vi "FPGA_main_sensorTest.vi"() -> ()   [LabVIEW 2020]
doc: "256-pt. MA filter in AI chain with control effort linearization based on feedback position."
uses:
  <vilib>/rvi/Emulation/niFpgaGetClockAttributes.vi
  <vilib>/rvi/Emulation/niFpgaSctlEmulationGetInTimedLoop.vi
  <vilib>/rvi/Emulation/niFpgaEmulationReportErrorSimple.vi
  <vilib>/rvi/eio/common/nirviEmuTemplateMethod_errors.vi
  <vilib>/rvi/Emulation/niFpgaEmulationIsFPGAContextNoSignature.vi
  <vilib>/rvi/errors/niFpgaSetErrorForExecOnDevCompSimple.vi
  <vilib>/rvi/eio/common/nirviEmuReportErrorAndStop.vi
  <vilib>/rvi/DataTransferAndStorage/Container/Common/niFpgaContainerGetUniqueNameForEmu.vi
  <vilib>/rvi/FIFO/Fifo_Resource/nirvififoEmulationSetSize.vi
  <vilib>/rvi/FIFO/Fifo_Resource/nirviFifoEmulationQueueMgr.vi
  <instcachedir>/0/nirviFifoEmulationQueueMgr_E5CAEC123FF24DC58D834DCA3CDAA9B5.lvgen/nirviFifoEmulationQueueMgr_E5CAEC123FF24DC58D834DCA3CDAA9B5_001.vi
  <vilib>/rvi/FIFO/Fifo_Resource/nirvififoEmulationDetermineInputValidOut.vi
  <vilib>/rvi/FIFO/Fifo_Resource/nirvififoEmulationCreateLock.vi
  <vilib>/rvi/Emulation/niFpgaProcessEmulError.vi
  <vilib>/rvi/FIFO/Fifo_Resource/nirvififoEmulationObtainLock.vi
  <vilib>/rvi/FIFO/Fifo_Resource/nirvififoEmulationReleaseLock.vi
  <vilib>/rvi/occurrence/nirviWaitOnOccurrenceBase.vi
  <vilib>/rvi/errors/nirviReportUnexpectedCaseInternalError.vi
  <vilib>/rvi/errors/nirviReportUnexpectedCaseInternalError (U32).vi
  <vilib>/rvi/Emulation/niFpgaCriticalErrorInLSC.vi
  <vilib>/Utility/error.llb/Clear Errors.vi
  <vilib>/eio/EIONode/EIONode.xnode
  <vilib>/rvi/DataTransferAndStorage/Container/XNode/niFpgaContainer.xnode
  <vilib>/rvi/FIFO/Fifo_Resource/nirvififoEmulationWrite.vi
  <vilib>/rvi/FIFO/Fifo_Resource/nirvififoEmulationRead.vi
  Components/FPGA functions/FPGA functions.lvlib
panel:
  out "AI LS filter Loop time [us]":u8
  out "Mod7 (NI 9222) AI":fxp<+/-,25,5>[](array[numeric])
  out "AI LS Loop time [us]":u8
  out "FPGA AI LS FIFO\nOverflow?":bool
  out "Mod8 (NI 9222) AI":fxp<+/-,25,5>[](array[numeric])
  out "AI HS filter Loop time [ticks]":u8
  out "FPGA AI HS FIFO\nOverflow?":bool
  out "AI HS Loop time [ticks]":u8
  # "1 tick = 25 ns"
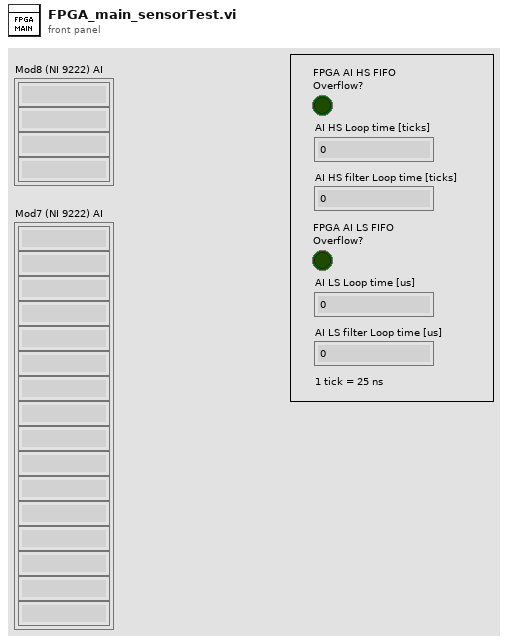
[diagram p1: front panel]
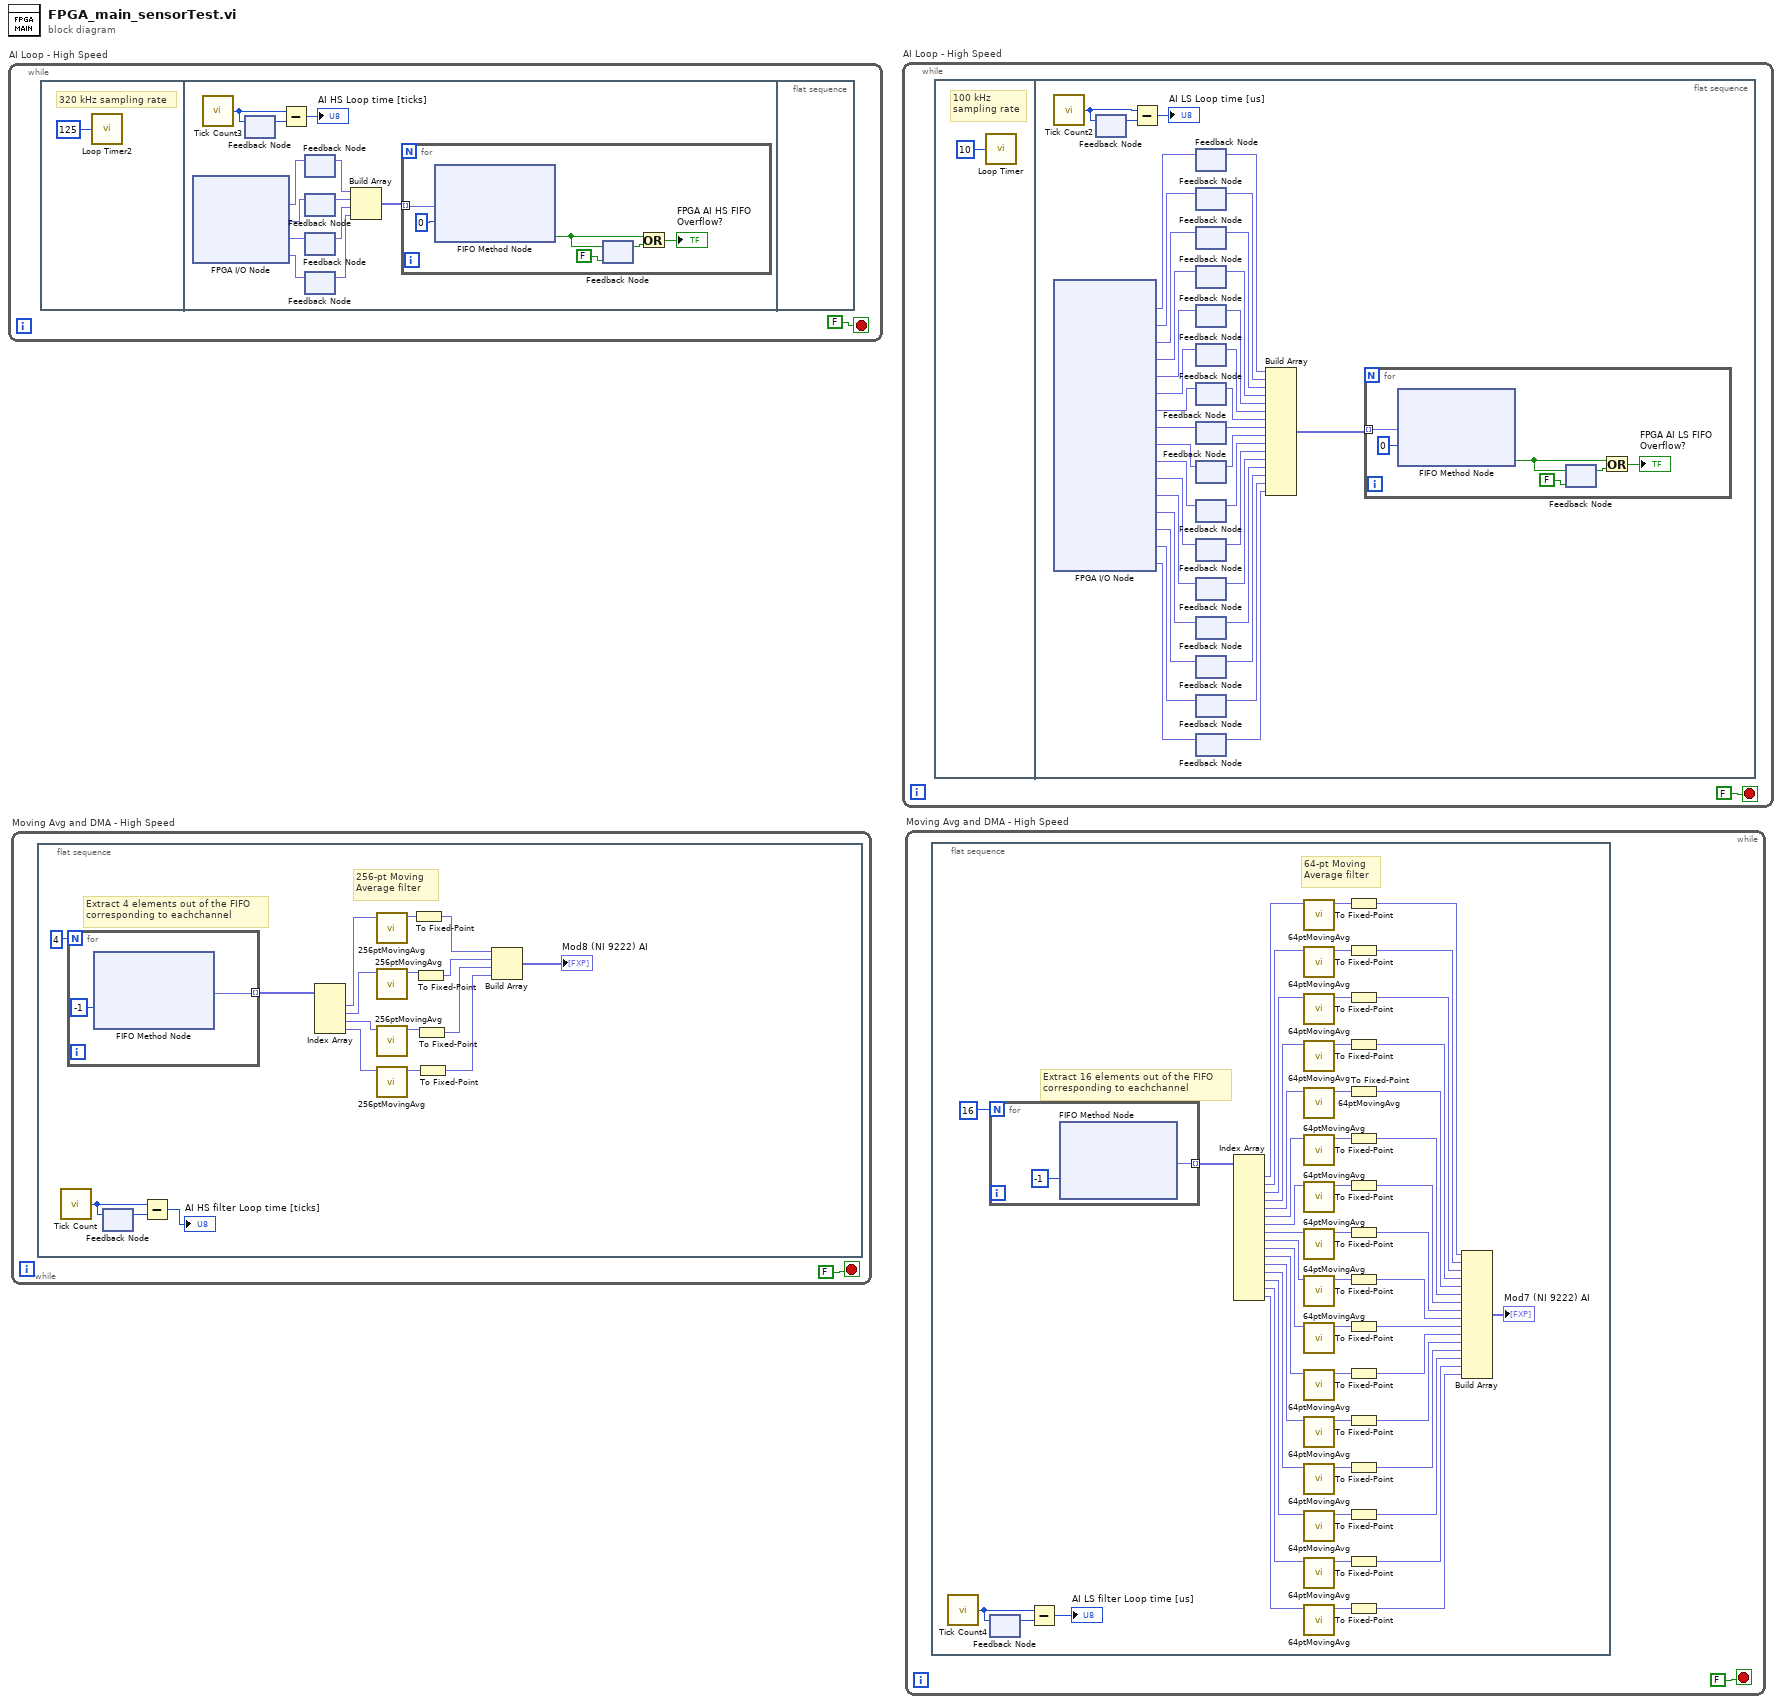
[diagram p0: block diagram]
diagram:
  n1 = while "AI Loop - High Speed" {
    stop <- FALSE stop-if-true
    n2 = flat-sequence {
      frame #0 {
        # "320 kHz sampling rate"
        n3 = call "Loop Timer2"("Count(Ticks)"=u8 125) -> ()  [unwired: 1 out]
      }
      frame #1 {
        n4 = xnode "FPGA I/O Node"() -> ("Mod8/AI0"=w9:fxp<+/-,24,5>, "Mod8/AI1"=w8:fxp<+/-,24,5>, "Mod8/AI2"=w7:fxp<+/-,24,5>, "Mod8/AI3"=w6:fxp<+/-,24,5>)  [unwired: 4 in, 4 out]
        n5 = call "Tick Count3"() -> ("Tick Count(Ticks)"=w14:u8)
        n6 = feedback #1() -> (w13:u8)  [unwired: 1 in]
        n7 = feedback-in #1(w14) -> ()
        n8 = Subtract(x=w14, y=w13) -> (x-y=→"AI HS Loop time [ticks]":u8)
        n9 = feedback-in #2(w9) -> ()
        n10 = feedback #2() -> (w10:fxp<+/-,24,5>)  [unwired: 1 in]
        n11 = feedback #3() -> (w5:fxp<+/-,24,5>)  [unwired: 1 in]
        n12 = feedback-in #3(w8) -> ()
        n13 = feedback #4() -> (w4:fxp<+/-,24,5>)  [unwired: 1 in]
        n14 = feedback-in #4(w7) -> ()
        n15 = feedback #5() -> (w3:fxp<+/-,24,5>)  [unwired: 1 in]
        n16 = feedback-in #5(w6) -> ()
        n17 = Build Array(w10, w5, w4, w3) -> (w11:fxp<+/-,24,5>[])
        n18 = for {
          tunnel: w11 -> [w19] mode=indexing
          n19 = xnode ("FIFO Method Node")("Element"=w19, "Timeout"=0) -> ("Timed Out?"=w16:bool)  [unwired: 1 in, 1 out]
          n20 = feedback-in #6(w16) -> ()
          n21 = feedback #6(FALSE ("Timed Out?")) -> (w17:bool)
          n22 = Or(x=w16, y=w17) -> (x .or. y?=→"FPGA AI HS FIFO\nOverflow?":bool)
        }
      }
      frame #2 {
      }
    }
  }
  n23 = while "Moving Avg and DMA - High Speed" {
    stop <- FALSE stop-if-true
    n24 = flat-sequence {
      frame #0 {
        # "256-pt Moving \nAverage filter"
        # "Extract 4 elements out of the FIFO \ncorresponding to eachchannel"
        n25 = call "Tick Count"() -> ("Tick Count(Ticks)"=w38:u8)
        n26 = for {
          N: 4 -> [_]
          tunnel: [w40] -> w35 mode=indexing
          n27 = xnode ("FIFO Method Node")("Timeout"=-1) -> ("Element"=w40:fxp<+/-,24,5>)  [unwired: 1 in, 2 out]
        }
        n28 = feedback #7() -> (w37:u8)  [unwired: 1 in]
        n29 = feedback-in #7(w38) -> ()
        n30 = Subtract(x=w38, y=w37) -> (x-y=→"AI HS filter Loop time [ticks]":u8)
        n31 = Index Array(array=w35) -> (element #1=w34:fxp<+/-,24,5>, element #2=w33:fxp<+/-,24,5>, element #3=w31:fxp<+/-,24,5>, element #4=w32:fxp<+/-,24,5>)  [unwired: 4 in]
        n32 = call "256ptMovingAvg.vi"("Raw input"=w34) -> ("Output"=w30:fxp<+/-,28,5>)  [unwired: 10 in]
        n33 = call "256ptMovingAvg.vi"("Raw input"=w33) -> ("Output"=w28:fxp<+/-,28,5>)  [unwired: 10 in]
        n34 = call "256ptMovingAvg.vi"("Raw input"=w31) -> ("Output"=w27:fxp<+/-,28,5>)  [unwired: 10 in]
        n35 = call "256ptMovingAvg.vi"("Raw input"=w32) -> ("Output"=w24:fxp<+/-,28,5>)  [unwired: 10 in]
        n36 = To Fixed-Point(number=w30) -> (fixed-point=w29:fxp<+/-,25,5>)  [unwired: 1 in]
        n37 = To Fixed-Point(number=w28) -> (fixed-point=w26:fxp<+/-,25,5>)  [unwired: 1 in]
        n38 = To Fixed-Point(number=w27) -> (fixed-point=w25:fxp<+/-,25,5>)  [unwired: 1 in]
        n39 = To Fixed-Point(number=w24) -> (fixed-point=w23:fxp<+/-,25,5>)  [unwired: 1 in]
        n40 = Build Array(w29, w26, w25, w23) -> (→"Mod8 (NI 9222) AI":fxp<+/-,25,5>[])
      }
    }
  }
  n41 = while "AI Loop - High Speed" {
    stop <- FALSE stop-if-true
    n42 = flat-sequence {
      frame #0 {
        # "100 kHz \nsampling rate"
        n43 = call "Loop Timer"("Count(uSec)"=u8 10 ("Count(Ticks)")) -> ()  [unwired: 1 out]
      }
      frame #1 {
        n44 = call "Tick Count2"() -> ("Tick Count(uSec)"=w79:u8)
        n45 = xnode "FPGA I/O Node"() -> ("Mod7/AI0"=w75:fxp<+/-,24,5>, "Mod7/AI1"=w74:fxp<+/-,24,5>, "Mod7/AI2"=w73:fxp<+/-,24,5>, "Mod7/AI3"=w72:fxp<+/-,24,5>, "Mod7/AI4"=w71:fxp<+/-,24,5>, "Mod7/AI5"=w70:fxp<+/-,24,5>, "Mod7/AI6"=w69:fxp<+/-,24,5>, "Mod7/AI7"=w68:fxp<+/-,24,5>, "Mod7/AI8"=w67:fxp<+/-,24,5>, "Mod7/AI9"=w66:fxp<+/-,24,5>, "Mod7/AI10"=w65:fxp<+/-,24,5>, "Mod7/AI11"=w64:fxp<+/-,24,5>, "Mod7/AI12"=w63:fxp<+/-,24,5>, "Mod7/AI13"=w62:fxp<+/-,24,5>, "Mod7/AI14"=w61:fxp<+/-,24,5>, "Mod7/AI15"=w60:fxp<+/-,24,5>)  [unwired: 16 in, 16 out]
        n46 = feedback #8() -> (w78:u8)  [unwired: 1 in]
        n47 = feedback-in #8(w79) -> ()
        n48 = Subtract(x=w79, y=w78) -> (x-y=→"AI LS Loop time [us]":u8)
        n49 = feedback #9() -> (w59:fxp<+/-,24,5>)  [unwired: 1 in]
        n50 = feedback-in #9(w75) -> ()
        n51 = feedback #10() -> (w58:fxp<+/-,24,5>)  [unwired: 1 in]
        n52 = feedback-in #10(w74) -> ()
        n53 = feedback #11() -> (w57:fxp<+/-,24,5>)  [unwired: 1 in]
        n54 = feedback-in #11(w73) -> ()
        n55 = feedback #12() -> (w56:fxp<+/-,24,5>)  [unwired: 1 in]
        n56 = feedback-in #12(w72) -> ()
        n57 = feedback #13() -> (w55:fxp<+/-,24,5>)  [unwired: 1 in]
        n58 = feedback-in #13(w71) -> ()
        n59 = feedback #14() -> (w54:fxp<+/-,24,5>)  [unwired: 1 in]
        n60 = feedback-in #14(w70) -> ()
        n61 = feedback #15() -> (w53:fxp<+/-,24,5>)  [unwired: 1 in]
        n62 = feedback-in #15(w69) -> ()
        n63 = feedback #16() -> (w52:fxp<+/-,24,5>)  [unwired: 1 in]
        n64 = feedback-in #16(w68) -> ()
        n65 = feedback #17() -> (w51:fxp<+/-,24,5>)  [unwired: 1 in]
        n66 = feedback-in #17(w67) -> ()
        n67 = feedback #18() -> (w50:fxp<+/-,24,5>)  [unwired: 1 in]
        n68 = feedback-in #18(w66) -> ()
        n69 = feedback #19() -> (w49:fxp<+/-,24,5>)  [unwired: 1 in]
        n70 = feedback-in #19(w65) -> ()
        n71 = feedback #20() -> (w48:fxp<+/-,24,5>)  [unwired: 1 in]
        n72 = feedback-in #20(w64) -> ()
        n73 = feedback #21() -> (w47:fxp<+/-,24,5>)  [unwired: 1 in]
        n74 = feedback-in #21(w63) -> ()
        n75 = feedback #22() -> (w46:fxp<+/-,24,5>)  [unwired: 1 in]
        n76 = feedback-in #22(w62) -> ()
        n77 = feedback #23() -> (w45:fxp<+/-,24,5>)  [unwired: 1 in]
        n78 = feedback-in #23(w61) -> ()
        n79 = feedback #24() -> (w44:fxp<+/-,24,5>)  [unwired: 1 in]
        n80 = feedback-in #24(w60) -> ()
        n81 = Build Array(w59, w58, w57, w56, w55, w54, w53, w52, w51, w50, w49, w48, w47, w46, w45, w44) -> (w76:fxp<+/-,24,5>[])
        n82 = for {
          tunnel: w76 -> [w80] mode=indexing
          n83 = xnode ("FIFO Method Node")("Element"=w80, "Timeout"=0) -> ("Timed Out?"=w82:bool)  [unwired: 1 in, 1 out]
          n84 = feedback-in #25(w82) -> ()
          n85 = feedback #25(FALSE ("Timed Out?")) -> (w83:bool)
          n86 = Or(x=w82, y=w83) -> (x .or. y?=→"FPGA AI LS FIFO\nOverflow?":bool)
        }
      }
    }
  }
  n87 = while "Moving Avg and DMA - High Speed" {
    stop <- FALSE stop-if-true
    n88 = flat-sequence {
      frame #0 {
        # "64-pt Moving \nAverage filter"
        # "Extract 16 elements out of the FIFO \ncorresponding to eachchannel"
        n89 = call "Tick Count4"() -> ("Tick Count(uSec)"=w139:u8)
        n90 = for {
          N: 16 -> [_]
          tunnel: [w141] -> w136 mode=indexing
          n91 = xnode ("FIFO Method Node")("Timeout"=-1) -> ("Element"=w141:fxp<+/-,24,5>)  [unwired: 1 in, 2 out]
        }
        n92 = feedback #26() -> (w138:u8)  [unwired: 1 in]
        n93 = feedback-in #26(w139) -> ()
        n94 = Subtract(x=w139, y=w138) -> (x-y=→"AI LS filter Loop time [us]":u8)
        n95 = Index Array(array=w136) -> (element #1=w133:fxp<+/-,24,5>, element #2=w132:fxp<+/-,24,5>, element #3=w131:fxp<+/-,24,5>, element #4=w130:fxp<+/-,24,5>, element #5=w129:fxp<+/-,24,5>, element #6=w128:fxp<+/-,24,5>, element #7=w127:fxp<+/-,24,5>, element #8=w126:fxp<+/-,24,5>, element #9=w125:fxp<+/-,24,5>, element #10=w124:fxp<+/-,24,5>, element #11=w123:fxp<+/-,24,5>, element #12=w122:fxp<+/-,24,5>, element #13=w121:fxp<+/-,24,5>, element #14=w120:fxp<+/-,24,5>, element #15=w119:fxp<+/-,24,5>, element #16=w118:fxp<+/-,24,5>)  [unwired: 16 in]
        n96 = call "64ptMovingAvg.vi"("Raw input"=w133) -> ("Output"=w117:fxp<+/-,28,5>)  [unwired: 10 in]
        n97 = call "64ptMovingAvg.vi"("Raw input"=w132) -> ("Output"=w116:fxp<+/-,28,5>)  [unwired: 10 in]
        n98 = call "64ptMovingAvg.vi"("Raw input"=w131) -> ("Output"=w115:fxp<+/-,28,5>)  [unwired: 10 in]
        n99 = call "64ptMovingAvg.vi"("Raw input"=w130) -> ("Output"=w114:fxp<+/-,28,5>)  [unwired: 10 in]
        n100 = call "64ptMovingAvg.vi"("Raw input"=w129) -> ("Output"=w113:fxp<+/-,28,5>)  [unwired: 10 in]
        n101 = call "64ptMovingAvg.vi"("Raw input"=w128) -> ("Output"=w112:fxp<+/-,28,5>)  [unwired: 10 in]
        n102 = call "64ptMovingAvg.vi"("Raw input"=w127) -> ("Output"=w111:fxp<+/-,28,5>)  [unwired: 10 in]
        n103 = call "64ptMovingAvg.vi"("Raw input"=w126) -> ("Output"=w110:fxp<+/-,28,5>)  [unwired: 10 in]
        n104 = call "64ptMovingAvg.vi"("Raw input"=w125) -> ("Output"=w109:fxp<+/-,28,5>)  [unwired: 10 in]
        n105 = call "64ptMovingAvg.vi"("Raw input"=w124) -> ("Output"=w108:fxp<+/-,28,5>)  [unwired: 10 in]
        n106 = call "64ptMovingAvg.vi"("Raw input"=w123) -> ("Output"=w107:fxp<+/-,28,5>)  [unwired: 10 in]
        n107 = call "64ptMovingAvg.vi"("Raw input"=w122) -> ("Output"=w106:fxp<+/-,28,5>)  [unwired: 10 in]
        n108 = call "64ptMovingAvg.vi"("Raw input"=w121) -> ("Output"=w105:fxp<+/-,28,5>)  [unwired: 10 in]
        n109 = call "64ptMovingAvg.vi"("Raw input"=w120) -> ("Output"=w104:fxp<+/-,28,5>)  [unwired: 10 in]
        n110 = call "64ptMovingAvg.vi"("Raw input"=w119) -> ("Output"=w103:fxp<+/-,28,5>)  [unwired: 10 in]
        n111 = call "64ptMovingAvg.vi"("Raw input"=w118) -> ("Output"=w102:fxp<+/-,28,5>)  [unwired: 10 in]
        n112 = To Fixed-Point(number=w117) -> (fixed-point=w135:fxp<+/-,25,5>)  [unwired: 1 in]
        n113 = To Fixed-Point(number=w116) -> (fixed-point=w101:fxp<+/-,25,5>)  [unwired: 1 in]
        n114 = To Fixed-Point(number=w115) -> (fixed-point=w100:fxp<+/-,25,5>)  [unwired: 1 in]
        n115 = To Fixed-Point(number=w114) -> (fixed-point=w99:fxp<+/-,25,5>)  [unwired: 1 in]
        n116 = To Fixed-Point(number=w113) -> (fixed-point=w98:fxp<+/-,25,5>)  [unwired: 1 in]
        n117 = To Fixed-Point(number=w112) -> (fixed-point=w97:fxp<+/-,25,5>)  [unwired: 1 in]
        n118 = To Fixed-Point(number=w111) -> (fixed-point=w96:fxp<+/-,25,5>)  [unwired: 1 in]
        n119 = To Fixed-Point(number=w110) -> (fixed-point=w95:fxp<+/-,25,5>)  [unwired: 1 in]
        n120 = To Fixed-Point(number=w109) -> (fixed-point=w94:fxp<+/-,25,5>)  [unwired: 1 in]
        n121 = To Fixed-Point(number=w108) -> (fixed-point=w93:fxp<+/-,25,5>)  [unwired: 1 in]
        n122 = To Fixed-Point(number=w107) -> (fixed-point=w92:fxp<+/-,25,5>)  [unwired: 1 in]
        n123 = To Fixed-Point(number=w106) -> (fixed-point=w91:fxp<+/-,25,5>)  [unwired: 1 in]
        n124 = To Fixed-Point(number=w105) -> (fixed-point=w90:fxp<+/-,25,5>)  [unwired: 1 in]
        n125 = To Fixed-Point(number=w104) -> (fixed-point=w89:fxp<+/-,25,5>)  [unwired: 1 in]
        n126 = To Fixed-Point(number=w103) -> (fixed-point=w88:fxp<+/-,25,5>)  [unwired: 1 in]
        n127 = To Fixed-Point(number=w102) -> (fixed-point=w87:fxp<+/-,25,5>)  [unwired: 1 in]
        n128 = Build Array(w135, w101, w100, w99, w98, w97, w96, w95, w94, w93, w92, w91, w90, w89, w88, w87) -> (→"Mod7 (NI 9222) AI":fxp<+/-,25,5>[])
      }
    }
  }
